vi "DWE Filter Data.vi"(11 "All Rows":string[][](array[string])) -> (2 "element":i32, 3 "new array":string[][](array[string]))   [LabVIEW 2014]
doc: "Filter data rows so that only those from the boards are kept. Boards output Command 0x60."
panel:
  out "subarray 2":i32[](array[numeric])
  out "deleted portion":string[](array[string])
  out "Locations":i32[][](array[numeric])
  out "size(s)":i32[](array[numeric])
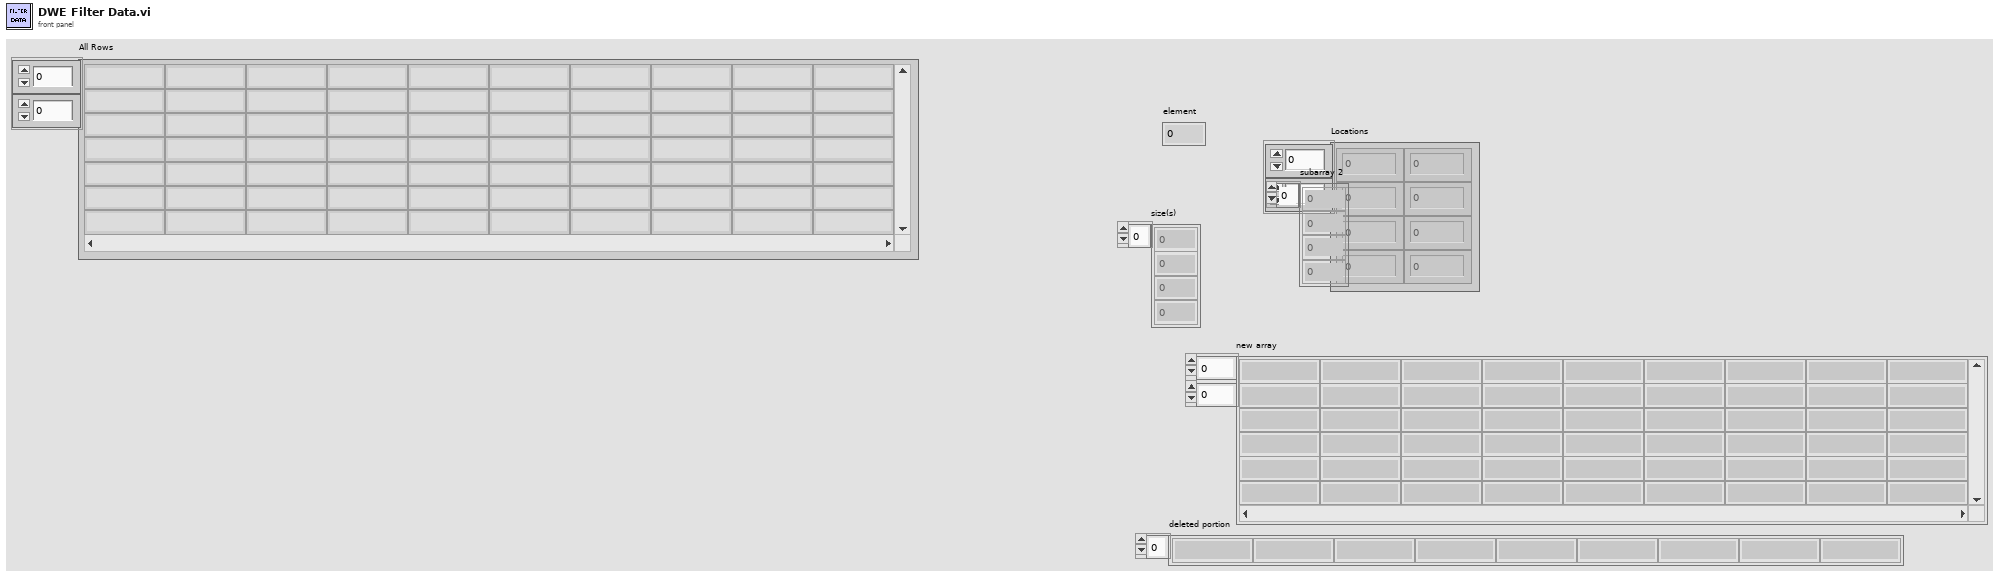
[diagram p1: front panel]
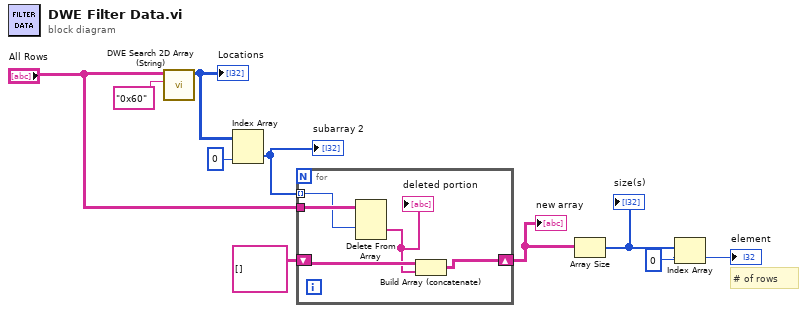
[diagram p0: block diagram]
diagram:
  # "# of rows"
  n1 = call "DWE Search 2D Array (String).vi"("Element"="0x60", "Array"="All Rows") -> ("Locations"=w3:i32[][])  [unwired: 9 in]
  "Locations" <- w3
  n2 = Index Array(array=w3, index (col)=0 ("disabled index (col)")) -> (element=w6:i32[])  [unwired: 1 in]
  "subarray 2" <- w6
  n3 = for {
    tunnel: w6 -> [w14] mode=indexing
    tunnel: "All Rows" -> [w15]
    shift-right: [w13] -> w2
    shift-left: string[][] [] -> [w12]
    n4 = Delete From Array(array=w15, index (row)=w14) -> (deleted portion=w11:string[])  [unwired: 2 in, 1 out]
    "deleted portion" <- w11
    n5 = Build Array (concatenate)(w12, w11) -> (w13:string[][])
  }
  "new array" <- w2
  n6 = Array Size(array=w2) -> (size(s)=w10:i32[])
  "size(s)" <- w10
  n7 = Index Array(array=w10, index=0) -> (element=→"element":i32)
